vi "Initialize.vi"() -> (14 "Fatal Error Out":T2, 15 "State Out":T1)   [LabVIEW 2017, in "ReadTag.xnode"]
doc: "Read Tag XNode script that initialises the node's state."
uses:
  ReadTag.xnode
  <vilib>/XNodeSupport/XNodeErrorCluster.ctl
  State.ctl
  <vilib>/XNodeSupport/NI_XNodeSupport.lvlib
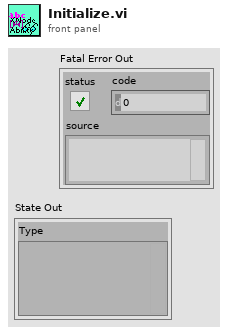
[diagram p1: front panel]
types:
  T1 = typedef "ReadTag.xnode/State.ctl" = cluster{"Type":variant}
  T2 = typedef "NI_XNodeSupport.lvlib/XNodeErrorCluster.ctl" = errorcluster
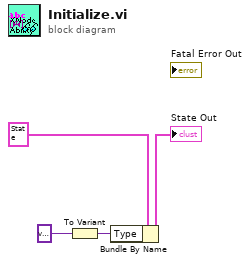
[diagram p0: block diagram]
diagram:
  n1 = To Variant(anything=variant ("Type")) -> (Variant=w1:variant)
  n2 = Bundle By Name(cluster=T1 {"Type"=variant} ("State Out"), "Type"=w1) -> (→"State Out":T1)
